vi "stop.vi"(11 "Experience ID":string="Test") -> (0 "error out":errorcluster={"status"=TRUE, "code"=2, "source"="incorrect path for Experience ID"})   [LabVIEW 2015]
uses:
  Configuration/Global_Configurations.vi
panel:
  # "Stop"
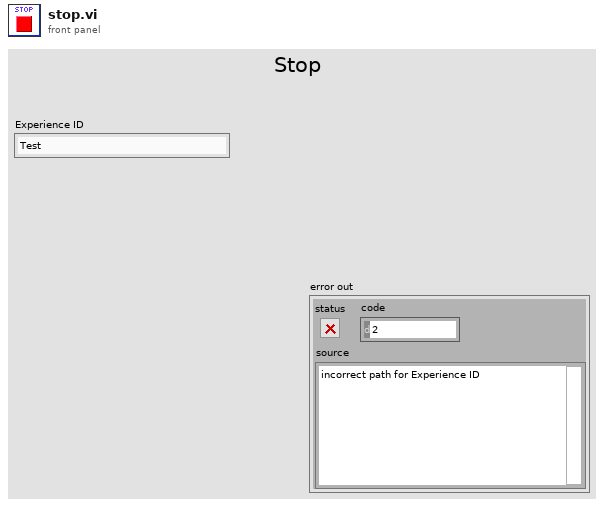
[diagram p1: front panel]
types:
  T1 = enum32{"Bad", "Idle", "Run top level", "Running"}
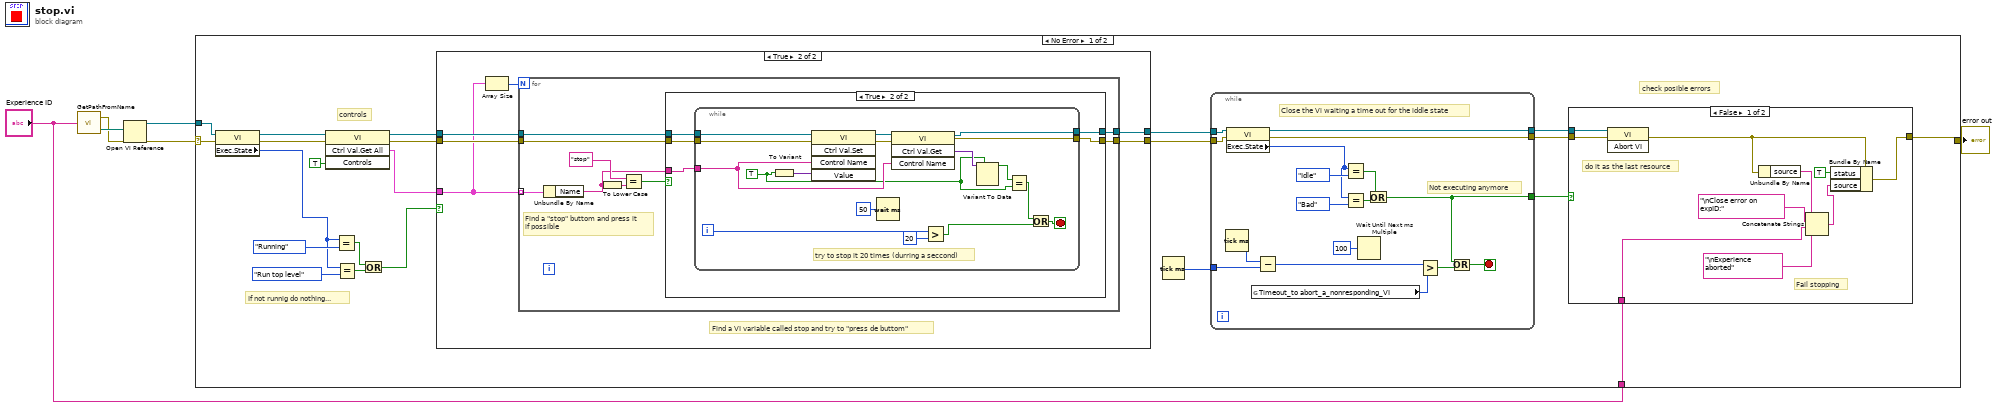
[diagram p0: block diagram]
diagram:
  n1 = call "GetPathFromName.vi"("Experience ID"="Experience ID") -> ("Error out"=w5:errorcluster, "VI_Path"=w6:path)
  n2 = Open VI Reference(vi path=w6, error in (no error)=w5) -> (vi reference=w2:refnum<vi>, error out=w3:errorcluster)  [unwired: 1 in, 3 out]
  n3 = case shown="No Error" w3 {
    selector: w3 -> [w17 w98]
    tunnel: [w14 w98] -> w4
    tunnel: w2 -> [w16 _]
    tunnel: "Experience ID" -> [w13 _]
    frame No Error {
      # "check posible errors"
      # "If not runnig do nothing..."
      # "controls"
      n4 = property class="VI"(reference=w16, error in=w17) -> (reference out=w22:refnum<vi>, error out=w21:errorcluster, "Exec.State"=w15:T1)
      n5 = invoke class="VI" method="Ctrl Val.Get All"(reference=w22, error in=w21, "Controls"=TRUE) -> (reference out=w23:refnum<vi>, error out=w20:errorcluster, "Get All Control Values Variant"=w19:cluster{"Name":string, "Variant Data":variant}[])  [unwired: 1 in, 1 out]
      n6 = Equal?(x=w15, y=T1."Running") -> (x = y?=w27:bool)
      n7 = Equal?(x=w15, y=T1."Run top level") -> (x = y?=w25:bool)
      n8 = Or(x=w27, y=w25) -> (x .or. y?=w18:bool)
      n9 = case shown="True" w18 {
        tunnel: w19 -> [_ w60]
        tunnel: w23 -> [w57 w64]
        tunnel: w20 -> [w58 w63]
        tunnel: [w58 w62] -> w12
        tunnel: [w57 w59] -> w11
        frame False {
        }
        frame True {
          # "Find a VI variable called stop and try to \"press de buttom\""
          n10 = Array Size(array=w60) -> (size(s)=w61:i32)
          n11 = for {
            N: w61 -> [_]
            tunnel: w60 -> [w73] mode=indexing
            tunnel: w64 -> [w71]
            tunnel: w63 -> [w70]
            tunnel: [w68] -> w62
            tunnel: [w65] -> w59
            # "Find a \"stop\" buttom and press it\nif possible"
            n12 = Unbundle By Name(w73) -> ("Name"=w66:string)
            n13 = To Lower Case(string=w66) -> (all lower case string=w67:string)
            n14 = Equal?(x="stop" ("y"), y=w67) -> (x = y?=w72:bool)
            n15 = case shown="True" w72 {
              tunnel: w71 -> [w74 w80]
              tunnel: w70 -> [w75 w79]
              tunnel: [w75 w78] -> w68
              tunnel: w66 -> [_ w77]
              tunnel: [w74 w76] -> w65
              frame False {
              }
              frame True {
                n16 = while {
                  tunnel: w80 -> [w95]
                  tunnel: w79 -> [w97]
                  tunnel: [w82] -> w78
                  tunnel: w77 -> [w87]
                  tunnel: [w81] -> w76
                  i -> [w93]
                  stop <- w94 stop-if-true
                  w84 = TRUE
                  # "try to stop it 20 times (durring a seccond)"
                  n17 = To Variant(anything=w84) -> (Variant=w96:variant)
                  n18 = invoke class="VI" method="Ctrl Val.Set"(reference=w95, error in=w97, "Control Name"=w87, "Value"=w96) -> (reference out=w89:refnum<vi>, error out=w88:errorcluster)  [unwired: 1 in, 3 out]
                  n19 = Wait (ms)(milliseconds to wait=u32 50) -> ()  [unwired: 1 out]
                  n20 = invoke class="VI" method="Ctrl Val.Get"(reference=w89, error in=w88, "Control Name"=w87) -> (reference out=w81:refnum<vi>, error out=w82:errorcluster, "Get Control Value Variant"=w86:variant)  [unwired: 1 in, 1 out]
                  n21 = Greater?(x=w93, y=20) -> (0:w91:bool)
                  n22 = Variant To Data(type=w84, Variant=w86) -> (data=w83:bool)  [unwired: 1 in, 1 out]
                  n23 = Equal?(x=w83, y=w84) -> (x = y?=w85:bool)
                  n24 = Or(x=w85, y=w91) -> (x .or. y?=w94:bool)
                }
              }
            }
          }
        }
      }
      n25 = Tick Count (ms)() -> (millisecond timer value=w10:u32)
      n26 = while {
        tunnel: w11 -> [w45]
        tunnel: [w35] -> w7
        tunnel: [w36] -> w9
        tunnel: [w30] -> w8
        tunnel: w10 -> [w38]
        tunnel: w12 -> [w29]
        stop <- w42 stop-if-true
        # "Not executing anymore"
        # "Close the Vi waiting a time out for the iddle state"
        n27 = Tick Count (ms)() -> (millisecond timer value=w37:u32)
        n28 = property class="VI"(reference=w45, error in=w29) -> (reference out=w35:refnum<vi>, error out=w36:errorcluster, "Exec.State"=w32:T1)
        n29 = global read "Global_Configurations.vi" "Timeout_to abort_a_nonresponding_VI"() -> (w39:u32)
        n30 = Subtract(x=w37, y=w38) -> (x-y=w40:u32)
        n31 = Equal?(x=w32, y=T1."Idle") -> (x = y?=w34:bool)
        n32 = Equal?(x=w32, y=T1."Bad") -> (x = y?=w31:bool)
        n33 = Wait Until Next ms Multiple(millisecond multiple=u32 100) -> ()  [unwired: 1 out]
        n34 = Or(x=w34, y=w31) -> (x .or. y?=w30:bool)
        n35 = Greater?(x=w40, y=w39) -> (0:w41:bool)
        n36 = Or(x=w30, y=w41) -> (x .or. y?=w42:bool)
      }
      n37 = case shown="False" w8 {
        tunnel: [w55 w56] -> w14
        tunnel: w9 -> [w47 w56]
        tunnel: w13 -> [w50 _]
        tunnel: w7 -> [w48 _]
        frame False {
          # "do it as the last resource"
          # "Fail stopping"
          n38 = invoke class="VI" method="Abort VI"(reference=w48, error in=w47) -> (error out=w49:errorcluster)  [unwired: 1 in, 2 out]
          n39 = Unbundle By Name(w49) -> ("source"=w52:string)
          n40 = Concatenate Strings(w52, "\nClose error on expID:" ("string"), w50, "\nExperience aborted" ("string")) -> (w53:string)
          n41 = Bundle By Name(cluster=w49, "status"=TRUE, "source"=w53) -> (w55:errorcluster)
        }
        frame True {
          # "ok"
        }
      }
    }
    frame Error {
    }
  }
  "error out" <- w4
